vi "Send Get All Controls at User Console.vi"(5 "Door Buttons":T1, 6 "Emergency":bool, 7 "Message Priority (Normal)":T4=enum."Normal", 8 "error in (no error)":errorcluster, 9 "Floor Selection":T2, 10 "Elevator Call":T3, 11 "Message Enqueuer":refnum<class "Message Enqueuer.lvclass">) -> (0 "error out":errorcluster, 3 "Message Enqueuer out":refnum<class "Message Enqueuer.lvclass">)   [LabVIEW 2019, in "Elevator Controller.lvlib" / "Get All Controls at User Console Msg.lvclass"]
doc: "This VI sends the message to an actor."
uses:
  Get All Controls at User Console Msg.lvclass
  <vilib>/ActorFramework/Message Enqueuer/Message Enqueuer.lvclass
  <vilib>/ActorFramework/Message Enqueuer/Message Priority.ctl
  Sim User Console Actor/Elevator Controller/Elevator Call -Cluster.ctl
  Sim User Console Actor/Elevator Controller/Floor Selection -Cluster.ctl
  Sim User Console Actor/Elevator Controller/Doors -Button.ctl
  C:/Program Files (x86)/National Instruments/LabVIEW 2019/vi.lib/ActorFramework/Message/Message.lvclass
  Get All Controls at User Console Msg.lvclass/Get All Controls at User Console Msg.ctl
  <vilib>/ActorFramework/Message Enqueuer/Message Enqueuer.lvclass/Message Enqueuer.ctl
  <vilib>/ActorFramework/Message Priority Queue/Priority Enqueue.vi
  Sim User Console Actor/Elevator Controller/Sim User Console Actor.lvclass
panel:
  # "Fourth Floor"
  # "Third Floor"
  # "Second Floor"
  # "First Floor"
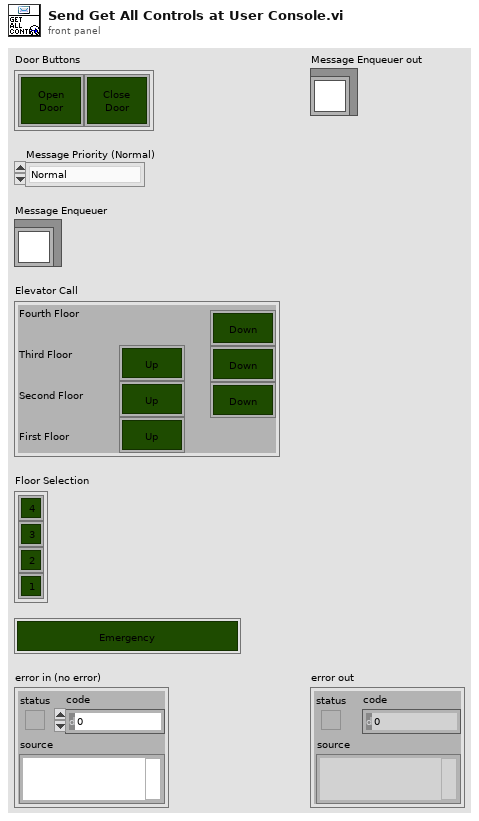
[diagram p1: front panel]
types:
  T1 = typedef "Sim User Console Actor.lvlib/Sim User Console Actor.lvclass/Doors -Button.ctl" = cluster{"Open Door":bool, "Close Door":bool}
  T2 = typedef "Sim User Console Actor.lvlib/Sim User Console Actor.lvclass/Floor Selection -Cluster.ctl" = cluster{"4":bool, "3":bool, "2":bool, "1":bool}
  T3 = typedef "Sim User Console Actor.lvlib/Sim User Console Actor.lvclass/Elevator Call -Cluster.ctl" = cluster{"Up 3":bool, "Up 2":bool, "Up 1":bool, "Down 4":bool, "Down 3":bool, "Down 2":bool}
  T4 = typedef "Actor Framework.lvlib/Message Enqueuer.lvclass/Message Priority.ctl" = enum16{"Low", "Normal", "High"}
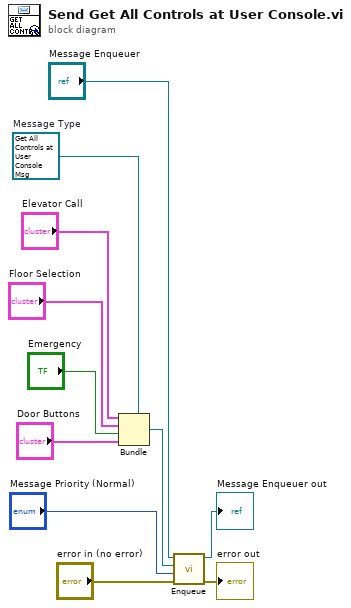
[diagram p0: block diagram]
diagram:
  w8 = refnum<class "Get All Controls at User Console Msg.lvclass"> refnum  # Message Type
  n1 = Bundle(cluster=w8, "Elevator Call", "Floor Selection", "Emergency", "Door Buttons") -> (w7:refnum<class "Get All Controls at User Console Msg.lvclass">)
  n2 = call <vilib>:"Enqueue.vi"("error in (no error)"="error in (no error)", "Message Priority (Normal)"="Message Priority (Normal)", "Message"=w7, "Message Enqueuer in"="Message Enqueuer") -> ("error out"=→"error out":errorcluster, "Message Enqueuer out"=→"Message Enqueuer out":refnum<class "Message Enqueuer.lvclass">)  [unwired: 6 in]
